vi "Autonomous Independent.vi"() -> ()   [LabVIEW 2013]
doc: "This VI is called when autonomous begins, and will automatically be terminated when autonomous ends. You can carry out timed or sensor driven robot movement independently without needing to return to the caller."
uses:
  Robot Global Data.vi
  <vilib>/addons/control/pid/pid.llb/PID (DBL).vi
  <vilib>/Rock Robotics/WPI/RobotDrive/WPI_RobotDriveGetSetRefNum.vi
  <vilib>/Rock Robotics/WPI/Joystick/WPI_JoystickGetSetRefNum.vi
  <vilib>/Rock Robotics/WPI/RobotDrive/WPI_RobotDriveArcadeDrive_Standard(NoSaturation).vi
  <vilib>/addons/control/pid/NI_PID_pid.lvlib
panel:
  in  "PID gains":T1={"proportional gain (Kc)"=1.0, "integral time (Ti, min)"=0.01, "derivative time (Td, min)"=0.0} {"derivative time (Td, min)" format="%.3f"; "integral time (Ti, min)" format="%.3f"; "proportional gain (Kc)" format="%.3f"}
  in  "Stop":bool
  in  "SP:":dbl(slide)=60.7843137254902 min=0.0 max=0.0 scale=0.0..100.0
  out "MV:":dbl(slide)=18.78965245852964 scale=-100.0..100.0
  out "Current Movement, for debugging":T2 {"Y Joystick Value" scale=1.0..-1.0; "X Joystick Value" scale=-1.0..1.0}
  in  "Array of robot movements":T3(array[cluster]) {"Y Joystick Value" scale=1.0..-1.0; "X Joystick Value" scale=-1.0..1.0}
  # "Be sure to right-click and choose Data Operations>>Make Current Value default if you want to save the array values with the VI"
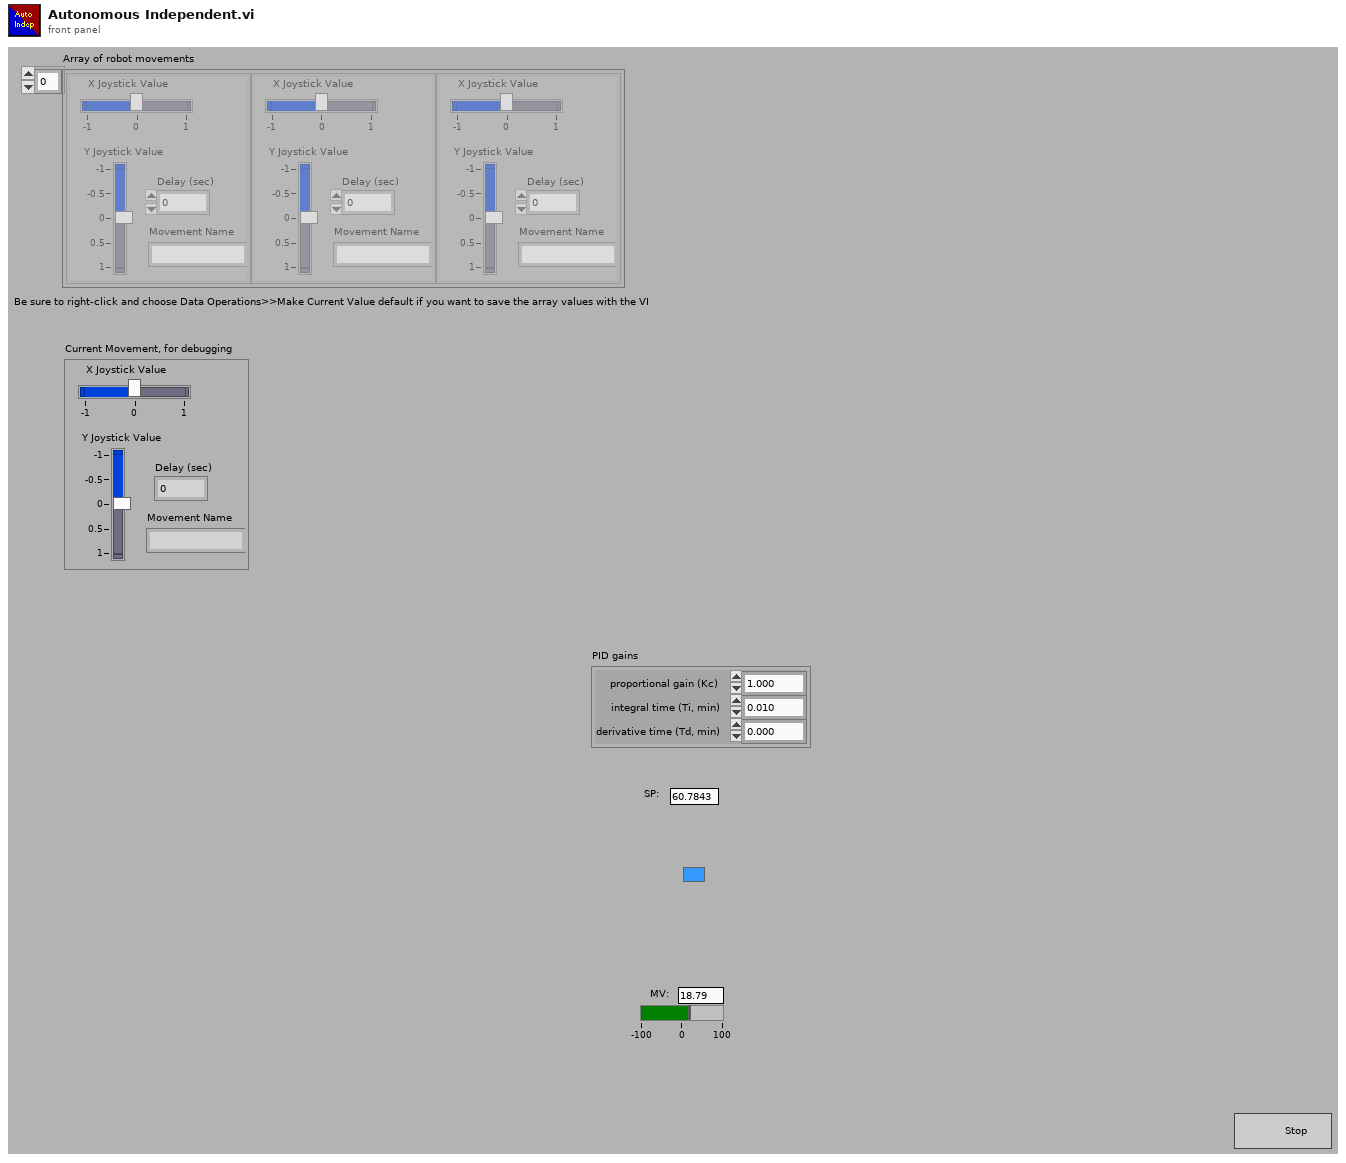
[diagram p1: front panel]
types:
  T1 = cluster{"proportional gain (Kc)":dbl, "integral time (Ti, min)":dbl, "derivative time (Td, min)":dbl}
  T2 = cluster{"X Joystick Value":dbl, "Y Joystick Value":dbl, "Delay (sec)":dbl, "Movement Name":string}
  T3 = cluster{"X Joystick Value":dbl, "Y Joystick Value":dbl, "Delay (sec)":dbl, "Movement Name":string}[]
  T4 = typedef "WPI_JoystickDevRef.ctl" = cluster{"Device":T5}
  T5 = typedef "WPI_JoystickDeviceEnum.ctl" = enum16{"USB 1", "USB 2", "USB 3", "USB 4", "Kinect 1", "Kinect 2"}
  T6 = typedef "WPI_EncoderDevRef.ctl" = cluster{"DevStatus":errorcluster, "EncoderIndex":T7, "CounterIndex":T8, "DistancePerCount":dbl, "Decoding Type":T9}
  T7 = typedef "FPGA_EncoderIdx.ctl" = enum8{"Enc 0", "Enc 1", "Enc 2", "Enc 3", "Invalid"}
  T8 = typedef "FPGA_CounterCtrSystemIndex.ctl" = enum8{"Ctr 0", "Ctr 1", "Ctr 2", "Ctr 3", "Ctr 4", "Ctr 5", "Ctr 6", "Ctr 7", "Invalid"}
  T9 = typedef "WPI_EncoderType.ctl" = enum16{"1x", "2x", "4x"}
  T10 = cluster{"axis 1 (x)":dbl, "axis 2 (y)":dbl, "axis 3 (throttle)":dbl, "axis 4":dbl, "axis 5":dbl, "axis 6":dbl}
  T11 = typedef "WPI_RobotDriveDevRef.ctl" = cluster{"DevStatus":errorcluster, "Motors[]":T12[], "Square Inputs":bool, "Max Output":dbl, "Isochronous":bool}
  T12 = typedef "WPI_MotorControlDeviceRef.ctl" = cluster{"DeviceStatus":errorcluster, "Type":enum16{"PWM", "CAN"}, "PWM":cluster{"Digital Module":T13, "PWM Channel":T14, "DeadBand":T15}, "CAN":cluster{"Device Number":u8, "Control Mode":T16, "Semaphore":T17, "Max Vout":dbl}, "Invert":bool, "TransformRef":T18, "InvTransformRef":T18}
  T13 = typedef "FPGA_TypedefDigitalModule.ctl" = enum16{"Digital Module 1", "Digital Module 2"}
  T14 = typedef "FPGA_DIOPWMChannel.ctl" = enum8{"PWM 1", "PWM 2", "PWM 3", "PWM 4", "PWM 5", "PWM 6", "PWM 7", "PWM 8", "PWM 9", "PWM 10", "Invalid"}
  T15 = typedef "WPI_PWMDeadband.ctl" = cluster{"Name":string, "maxPositivePwm":i32, "minPositivePwm":i32, "centerPwm":i32, "maxNegativePwm":i32, "minNegativePwm":i32, "angularRange":u16}
  T16 = typedef "WPI_CANJaguar_ControlMode.ctl" = enum8{"Percent VBus", "Current", "Speed", "Position", "Voltage"}
  T17 = typedef "Semaphore RefNum" = refnum<k1>
  T18 = typedef "WPI_PWMTransform_ConPane.ctl" = refnum<vi>
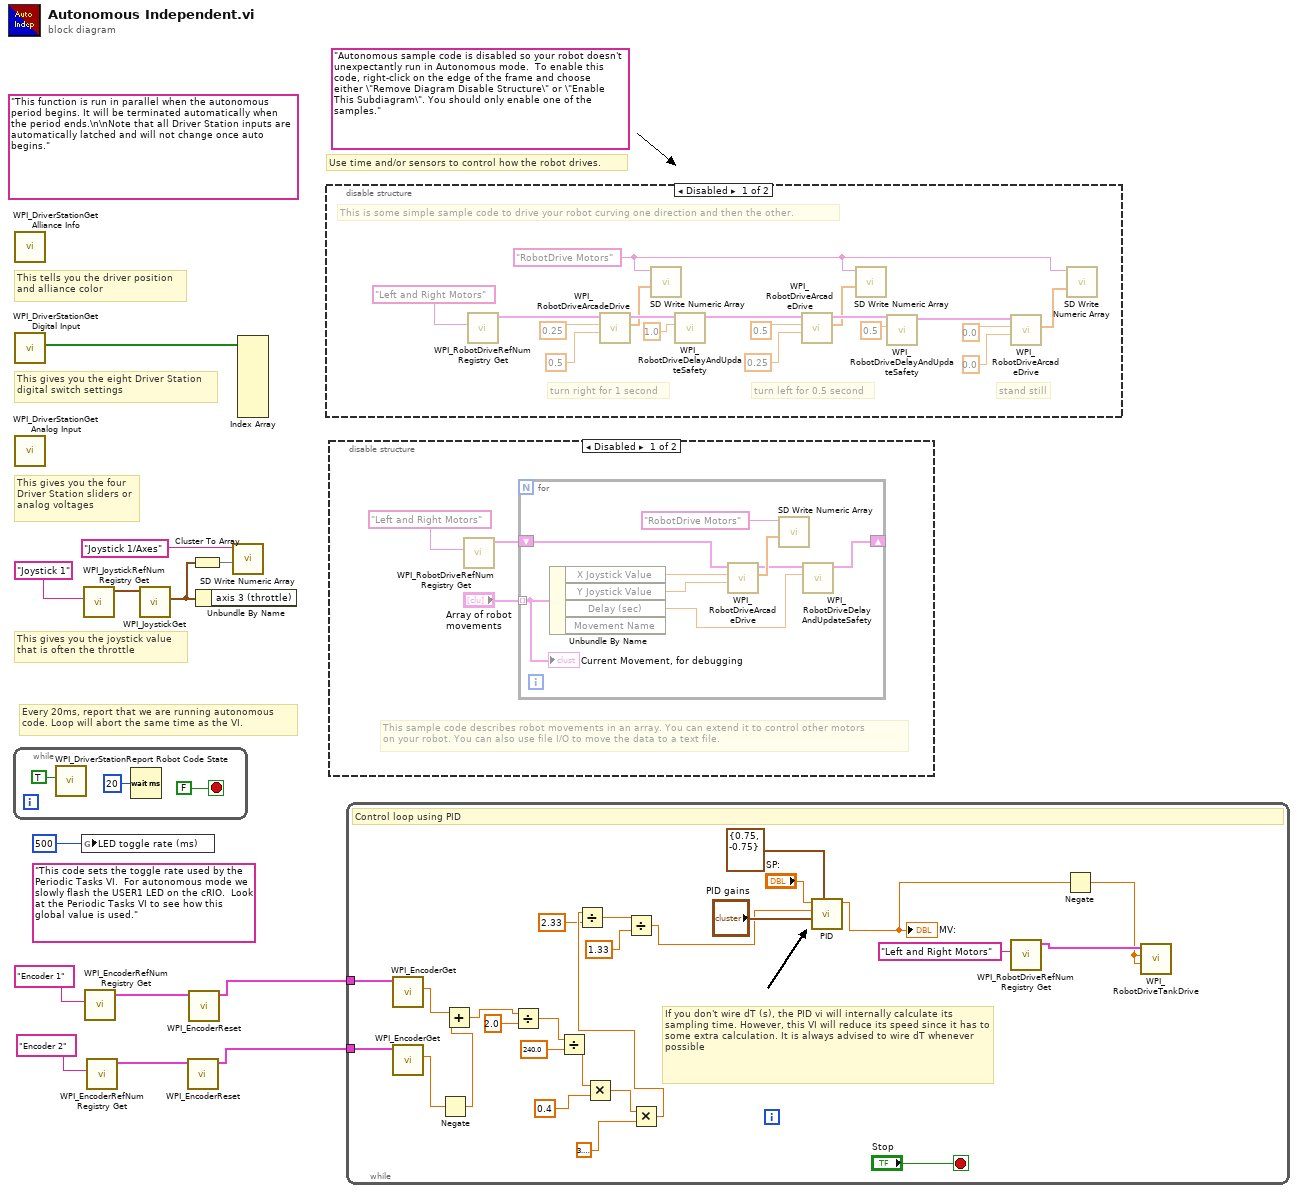
[diagram p0: block diagram]
diagram:
  (unwired) "This code sets the toggle rate used by the Periodic Tasks VI.  For autonomous mode we slowly flash the USER1 LED on the cRIO.  Look at the Periodic Tasks VI to see how this global value is used."
  (unwired) "Autonomous sample code is disabled so your robot doesn't unexpectantly run in Autonomous mode.  To enable this code, right-click on the edge of the frame and choose either \"Remove Diagram Disable Structure\" or \"Enable This Subdiagram\". You should only enable one of the samples."
  (unwired) "This function is run in parallel when the autonomous period begins. It will be terminated automatically when the period ends.\n\nNote that all Driver Station inputs are automatically latched and will not change once auto begins."
  # "Every 20ms, report that we are running autonomous\ncode. Loop will abort the same time as the VI."
  # "This gives you the joystick value\nthat is often the throttle"
  # "Use time and/or sensors to control how the robot drives."
  # "This tells you the driver position\nand alliance color"
  # "This gives you the eight Driver Station\ndigital switch settings"
  # "This gives you the four\nDriver Station sliders or\nanalog voltages"
  n1 = while {
    stop <- FALSE stop-if-true
    n2 = call <vilib>:"WPI_DriverStationReport Robot Code State.vi"("Autonomous"=TRUE) -> ()  [unwired: 10 in, 1 out]
    n3 = Wait (ms)(milliseconds to wait=u32 20) -> ()  [unwired: 1 out]
  }
  n4 = call <vilib>:"WPI_DriverStationGet Alliance Info.vi"() -> ()  [unwired: 12 out]
  n5 = call <vilib>:"WPI_DriverStationGet Digital Input.vi"() -> ("Driver Station Digital Input (1-8)"=w13:bool[])  [unwired: 11 out]
  n6 = call <vilib>:"WPI_DriverStationGet Analog Input.vi"() -> ()  [unwired: 12 out]
  n7 = global write "Robot Global Data.vi" "LED toggle rate (ms)"(u32 500 ("LED ms toggle rate")) -> ()
  n8 = call <vilib>:"WPI_JoystickRefNum Registry Get.vi"("refnum name"="Joystick 1") -> ("JoystickDevRef"=w11:T4)  [unwired: 1 in, 9 out]
  n9 = call <vilib>:"WPI_EncoderRefNum Registry Get.vi"("refnum name"="Encoder 1") -> ("EncoderDevRef"=w3:T6)  [unwired: 9 in, 1 out]
  n10 = call <vilib>:"WPI_EncoderRefNum Registry Get.vi"("refnum name"="Encoder 2") -> ("EncoderDevRef"=w4:T6)  [unwired: 9 in, 1 out]
  n11 = call <vilib>:"WPI_JoystickGet.vi"("JoystickDevRef"=w11) -> ("Axes"=w8:T10)  [unwired: 1 in, 5 out]
  n12 = call <vilib>:"WPI_EncoderReset.vi"("EncoderDevRef"=w4) -> ("EncoderDevRef"=w1:T6)  [unwired: 9 in, 1 out]
  n13 = call <vilib>:"WPI_EncoderReset.vi"("EncoderDevRef"=w3) -> ("EncoderDevRef"=w2:T6)  [unwired: 9 in, 1 out]
  n14 = Cluster To Array(cluster=w8) -> (array=w9:dbl[])
  n15 = Unbundle By Name(w8) -> ()  [unwired: 1 out]
  n16 = call <vilib>:"SD Write Numeric Array.vi"("Numeric Array"=w9, "Name"="Joystick 1/Axes") -> ()  [unwired: 8 in, 2 out]
  n17 = Index Array(array=w13) -> ()  [unwired: 8 in, 8 out]
  n18 = disable-structure shown="Disabled" {
    frame Disabled {
      w17 = "RobotDrive Motors" ("Name")
      # "This is some simple sample code to drive your robot curving one direction and then the other."
      # "stand still"
      # "turn left for 0.5 second"
      # "turn right for 1 second"
      n19 = call <vilib>:"WPI_RobotDriveRefNum Registry Get.vi"("refnum name"="Left and Right Motors") -> ("RobotDriveDevRef"=w21:T11)  [unwired: 1 in, 9 out]
      n20 = call-poly <vilib>:"WPI_RobotDriveArcadeDrive.vi"("Y axis value"=0.5 ("X axis value"), "X axis value"=0.25, "RobotDriveDevRef"=w21) -> ("Motor Values"=w20:dbl[], "RobotDriveDevRef"=w28:T11)  [unwired: 1 in, 6 out]
      n21 = call <vilib>:"SD Write Numeric Array.vi"("Numeric Array"=w20, "Name"=w17) -> ()  [unwired: 8 in, 2 out]
      n22 = call <vilib>:"WPI_RobotDriveDelayAndUpdateSafety.vi"("Delay (s)"=1.0, "RobotDriveDevRef"=w28) -> ("RobotDriveDevRef 2"=w27:T11)  [unwired: 8 in, 1 out]
      n23 = call-poly <vilib>:"WPI_RobotDriveArcadeDrive.vi"("Y axis value"=0.25 ("X axis value"), "X axis value"=0.5, "RobotDriveDevRef"=w27) -> ("Motor Values"=w19:dbl[], "RobotDriveDevRef"=w26:T11)  [unwired: 1 in, 6 out]
      n24 = call <vilib>:"SD Write Numeric Array.vi"("Numeric Array"=w19, "Name"=w17) -> ()  [unwired: 8 in, 2 out]
      n25 = call <vilib>:"WPI_RobotDriveDelayAndUpdateSafety.vi"("Delay (s)"=0.5, "RobotDriveDevRef"=w26) -> ("RobotDriveDevRef 2"=w25:T11)  [unwired: 8 in, 1 out]
      n26 = call-poly <vilib>:"WPI_RobotDriveArcadeDrive.vi"("Y axis value"=0.0 ("X axis value"), "X axis value"=0.0, "RobotDriveDevRef"=w25) -> ("Motor Values"=w18:dbl[])  [unwired: 1 in, 7 out]
      n27 = call <vilib>:"SD Write Numeric Array.vi"("Numeric Array"=w18, "Name"=w17) -> ()  [unwired: 8 in, 2 out]
    }
    frame Enabled {
    }
  }
  n28 = disable-structure shown="Disabled" {
    frame Disabled {
      # "This sample code describes robot movements in an array. You can extend it to control other motors\non your robot. You can also use file I/O to move the data to a text file."
      n29 = call <vilib>:"WPI_RobotDriveRefNum Registry Get.vi"("refnum name"="Left and Right Motors") -> ("RobotDriveDevRef"=w36:T11)  [unwired: 1 in, 9 out]
      n30 = for {
        shift-right: [w42] -> _
        shift-left: w36 -> [w43]
        tunnel: "Array of robot movements" -> [w38] mode=indexing
        n31 = Unbundle By Name(w38) -> ("X Joystick Value"=w41:dbl, "Y Joystick Value"=w40:dbl, "Delay (sec)"=w39:dbl)  [unwired: 1 out]
        n32 = call-poly <vilib>:"WPI_RobotDriveArcadeDrive.vi"("Y axis value"=w40, "X axis value"=w41, "RobotDriveDevRef"=w43) -> ("Motor Values"=w45:dbl[], "RobotDriveDevRef"=w44:T11)  [unwired: 1 in, 6 out]
        n33 = call <vilib>:"SD Write Numeric Array.vi"("Numeric Array"=w45, "Name"="RobotDrive Motors") -> ()  [unwired: 8 in, 2 out]
        n34 = call <vilib>:"WPI_RobotDriveDelayAndUpdateSafety.vi"("Delay (s)"=w39, "RobotDriveDevRef"=w44) -> ("RobotDriveDevRef 2"=w42:T11)  [unwired: 8 in, 1 out]
        "Current Movement, for debugging" <- w38
      }
    }
    frame Enabled {
    }
  }
  n35 = while {
    tunnel: w2 -> [w70]
    tunnel: w1 -> [w69]
    stop <- "Stop" stop-if-true
    # "If you don't wire dT (s), the PID vi will internally calculate its sampling time. However, this VI will reduce its speed since it has to some extra calculation. It is always advised to wire dT whenever possible"
    # "Control loop using PID"
    n36 = call <vilib>:"WPI_EncoderGet.vi"("EncoderDevRef"=w70) -> ("Distance"=w68:dbl)  [unwired: 5 in, 5 out]
    n37 = call <vilib>:"WPI_EncoderGet.vi"("EncoderDevRef"=w69) -> ("Distance"=w55:dbl)  [unwired: 5 in, 5 out]
    n38 = Negate(x=w55) -> (-x=w54:dbl)
    n39 = Add(x=w68, y=w54) -> (x+y=w66:dbl)
    n40 = Divide(x=w66, y=2.0) -> (x/y=w56:dbl)
    n41 = Divide(x=w56, y=240.0) -> (x/y=w64:dbl)
    n42 = Multiply(x=w64, y=0.4) -> (x*y=w61:dbl)
    n43 = Multiply(x=w61, y=3.141592653589793) -> (x*y=w53:dbl)
    n44 = Divide(x=w53, y=2.33) -> (x/y=w48:dbl)
    n45 = Divide(x=w48, y=1.33) -> (x/y=w49:dbl)
    n46 = call-poly <vilib>:"PID.vi"("output range"=cluster{"output high":dbl, "output low":dbl} {"output high"=0.75, "output low"=-0.75}, "PID gains"="PID gains", "process variable"=w49, "setpoint"="SP:") -> ("output"=w50:dbl)  [unwired: 6 in, 1 out]
    "MV:" <- w50
    n47 = call <vilib>:"WPI_RobotDriveRefNum Registry Get.vi"("refnum name"="Left and Right Motors") -> ("RobotDriveDevRef"=w57:T11)  [unwired: 9 in, 1 out]
    n48 = Negate(x=w50) -> (-x=w51:dbl)
    n49 = call <vilib>:"WPI_RobotDriveTankDrive.vi"("Right axis value"=w51, "Left axis value"=w51, "RobotDriveDevRef"=w57) -> ()  [unwired: 6 in, 3 out]
  }
